vi "4155C Sample Config SMUs v2.0.vi"(4 "Sample - Probe 4":u32(ring)=3 items=["SMU1  ", "SMU2  ", "SMU3  ", "SMU4  ", "SMU5  ", "SMU6  "], 5 "Sample - Drain":u32(ring)=1 items=["SMU1  ", "SMU2  ", "SMU3  ", "SMU4  ", "SMU5  ", "SMU6  "], 6 "Sample - Gate":u32(ring)=2 items=["SMU1  ", "SMU2  ", "SMU3  ", "SMU4  ", "SMU5  ", "SMU6  "], 7 "Sample - Source/Common":u32(ring) items=["SMU1  ", "SMU2  ", "SMU3  ", "SMU4  ", "SMU5  ", "SMU6  "], 8 "error in (no error)":errorcluster, 9 "Gate Standby":bool, 10 "Drain Standby":bool, 11 "VISA resource name in":refnum<visa-resource-name>) -> (0 "error out":errorcluster, 3 "VISA Resource Name out":refnum<visa-resource-name>)   [LabVIEW 2016]
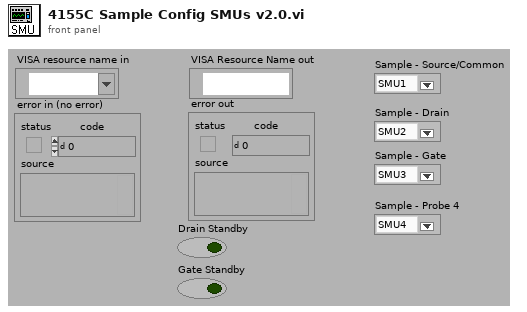
[diagram p1: front panel]
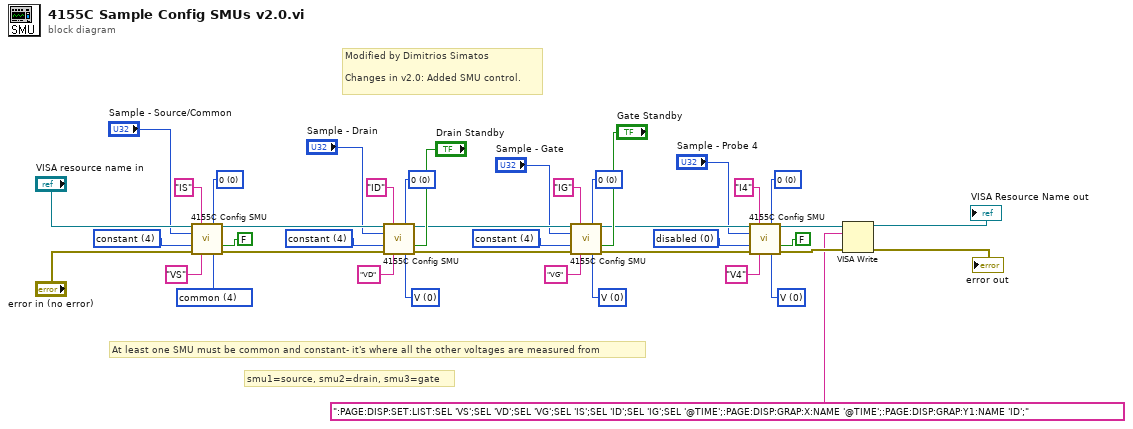
[diagram p0: block diagram]
diagram:
  w18 = u32 0 items=["V  ", "I  ", "V pulse  ", "I pulse  ", "  common  "] ("mode")
  w19 = u32 0 items=["0  ", "10K Ohms  ", "100K Ohms  ", "1M Ohms  "] ("series resistance *")
  w21 = u32 0 items=["disabled  ", "VAR1  ", "VAR2  ", "VAR1'  ", "constant  "] ("function")
  w24 = u32 0 items=["V  ", "I  ", "V pulse  ", "I pulse  ", "  common  "] ("mode")
  w25 = u32 0 items=["0  ", "10K Ohms  ", "100K Ohms  ", "1M Ohms  "] ("series resistance *")
  w27 = u32 4 items=["disabled  ", "VAR1  ", "VAR2  ", "VAR1'  ", "constant  "] ("function")
  w30 = u32 0 items=["V  ", "I  ", "V pulse  ", "I pulse  ", "  common  "] ("mode")
  w31 = u32 0 items=["0  ", "10K Ohms  ", "100K Ohms  ", "1M Ohms  "] ("series resistance *")
  w33 = u32 4 items=["disabled  ", "VAR1  ", "VAR2  ", "VAR1'  ", "constant  "] ("function")
  w36 = u32 4 items=["V  ", "I  ", "V pulse  ", "I pulse  ", "  common  "] ("mode")
  w37 = u32 0 items=["0  ", "10K Ohms  ", "100K Ohms  ", "1M Ohms  "] ("series resistance *")
  w39 = u32 4 items=["disabled  ", "VAR1  ", "VAR2  ", "VAR1'  ", "constant  "] ("function")
  # "Modified by Dimitrios Simatos\n\nChanges in v2.0: Added SMU control."
  # "smu1=source, smu2=drain, smu3=gate"
  # "At least one SMU must be common and constant- it's where all the other voltages are measured from"
  n1 = call "4155C Config SMU.vi"("VISA session"="VISA resource name in", "I name (max 6 chars)"="IS", "series resistance *"=w37, "unit to configure"="Sample - Source/Common", "function"=w39, "standby"=FALSE, "error in (no error)"="error in (no error)", "V name (max 6 chars)"="VS", "mode"=w36) -> ("dup VISA resource name"=w15:refnum<visa-resource-name>, "error out"=w14:errorcluster)  [unwired: 5 in]
  n2 = call "4155C Config SMU.vi"("VISA session"=w15, "I name (max 6 chars)"="ID", "series resistance *"=w31, "unit to configure"="Sample - Drain", "function"=w33, "standby"="Drain Standby", "error in (no error)"=w14, "V name (max 6 chars)"="VD", "mode"=w30) -> ("dup VISA resource name"=w12:refnum<visa-resource-name>, "error out"=w13:errorcluster)  [unwired: 5 in]
  n3 = call "4155C Config SMU.vi"("VISA session"=w12, "I name (max 6 chars)"="IG", "series resistance *"=w25, "unit to configure"="Sample - Gate", "function"=w27, "standby"="Gate Standby", "error in (no error)"=w13, "V name (max 6 chars)"="VG", "mode"=w24) -> ("dup VISA resource name"=w11:refnum<visa-resource-name>, "error out"=w10:errorcluster)  [unwired: 5 in]
  n4 = call "4155C Config SMU.vi"("VISA session"=w11, "I name (max 6 chars)"="I4", "series resistance *"=w19, "unit to configure"="Sample - Probe 4", "function"=w21, "standby"=FALSE, "error in (no error)"=w10, "V name (max 6 chars)"="V4", "mode"=w18) -> ("dup VISA resource name"=w9:refnum<visa-resource-name>, "error out"=w8:errorcluster)  [unwired: 5 in]
  n5 = VISA Write(VISA resource name=w9, write buffer=":PAGE:DISP:SET:LIST:SEL 'VS';SEL 'VD';SEL 'VG';SEL 'IS';SEL 'ID';SEL 'IG';SEL '@TIME';:PAGE:DISP:GRAP:X:NAME '@TIME';:PAGE:DISP:GRAP:Y1:NAME 'ID';" ("write buffer (\"\")"), error in (no error)=w8) -> (VISA resource name out=→"VISA Resource Name out":refnum<visa-resource-name>, error out=→"error out":errorcluster)  [unwired: 1 out]
